vi "获取规格清单.vi"(7 "父类":string, 8 "error in (no error)":errorcluster caption="错误输入（无错误）", 9 "Folder Path":path caption="文件夹路径", 11 "规格 输入":refnum<class "规格.lvclass">) -> (0 "error out":errorcluster caption="错误输出", 1 "清单名称":string[](array[string]), 2 "规格":refnum<class>[](array[class]), 3 "规格 输出":refnum<class "规格.lvclass">)   [LabVIEW 2016, in "规格.lvclass"]
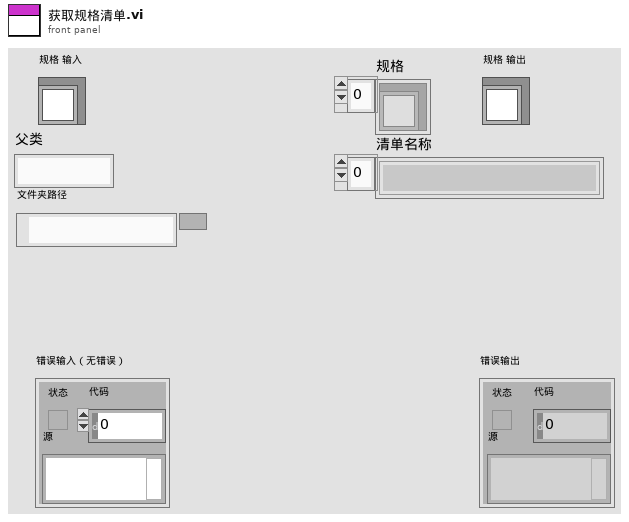
[diagram p1: front panel]
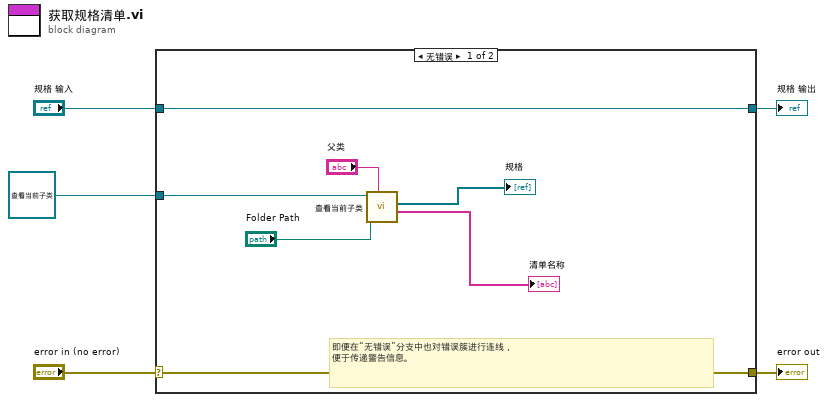
[diagram p0: block diagram]
diagram:
  n1 = case shown="无错误" "error in (no error)" {
    selector: "error in (no error)" -> [w11 w14]
    tunnel: [w11 w14] -> w4
    tunnel: [w12 w13] -> w2
    tunnel: "规格 输入" -> [w12 w13]
    tunnel: refnum<class "查看当前子类.lvclass"> refnum ("查看当前子类.lvclass") -> [w9 _]
    frame No Error {
      # "即便在“无错误”分支中也对错误簇进行连线，\n便于传递警告信息。"
      n2 = call-dynamic "查看当前子类.vi"("父类"="父类", "Folder Path"="Folder Path", "查看当前子类 输入"=w9) -> ("清单名称"=→"清单名称":string[], "数组"=→"规格":refnum<class>[])  [unwired: 5 in, 2 out]
    }
    frame Error {
    }
  }
  "error out" <- w4
  "规格 输出" <- w2
